vi "外设配置对话框.vi"() -> ()   [LabVIEW 2016, in "斯坦道氟化物.lvlib"]
uses:
  <vilib>/Utility/miscctls.llb/LVPointTypeDef.ctl
panel:
  out "选项卡控件":enum32{"V3 A版", "V3 B版"}(tab)
  in  "A版外设配置":T1 {"阀方向" items=["顺时针", "逆时针", "就近"]; "总氮x公式0" items=["0", "1"]; "光谱仪类型" items=["1型", "2型", "3型", "2型氙灯联控"]; "泵阀量" items=["9通"=9, "10通"=10, "12通"=12]; "泵类型" items=["1型", "2型", "sy04型+旋转阀"]}
  in  "B版外设配置":T2 {"阀型号" items=["垦拓10通阀"]; "总氮x公式0" items=["0", "1"]; "光谱仪类型" items=["1型", "2型", "3型", "2型氙灯联控"]; "泵阀量" items=["9通"=9, "10通"=10, "12通"=12]; "泵类型" items=["润泽注射泵", "垦拓注射泵"]}
  in  "关闭":bool
  in  "保存":bool
  in  "读取":bool
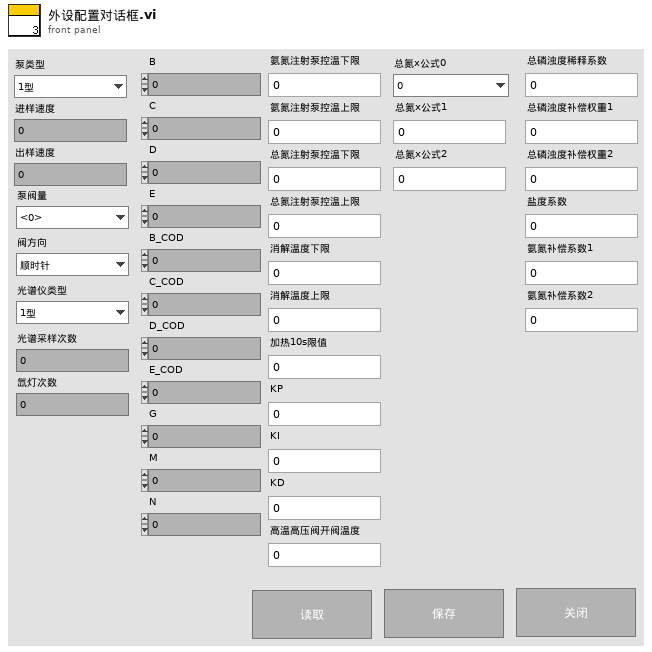
[diagram p1: front panel]
types:
  T1 = typedef "斯坦道氟化物.lvlib/V3 A版外设参数.ctl" = cluster{"泵类型":u8, "进样速度":u32, "出样速度":u32, "泵阀量":u8, "阀方向":u8, "光谱仪类型":u8, "光谱采样次数":u8, "氙灯次数":u8, "B":u16, "C":u16, "D":u16, "E":u16, "B_COD":u16, "C_COD":u16, "D_COD":u16, "E_COD":u16, "G":u16, "M":u16, "N":u16, "氨氮注射泵控温下限":sgl, "氨氮注射泵控温上限":sgl, "总氮注射泵控温下限":sgl, "总氮注射泵控温上限":sgl, "消解温度下限":sgl, "消解温度上限":sgl, "加热10s限值":sgl, "KP":sgl, "KI":sgl, "KD":sgl, "高温高压阀开阀温度":sgl, "总氮x公式0":u8, "总氮x公式1":sgl, "总氮x公式2":sgl, "总磷浊度稀释系数":sgl, "总磷浊度补偿权重1":sgl, "总磷浊度补偿权重2":sgl, "盐度系数":sgl, "氨氮补偿系数1":sgl, "氨氮补偿系数2":sgl}
  T2 = typedef "斯坦道氟化物.lvlib/V3 B版外设参数.ctl" = cluster{"泵类型":u8, "注射泵正常速度":u32, "注射泵慢速":u32, "泵阀量":u8, "阀型号":u8, "光谱仪类型":u8, "光谱采样次数":u8, "氙灯次数":u8, "B":u16, "C":u16, "D":u16, "E":u16, "B_COD":u16, "C_COD":u16, "D_COD":u16, "E_COD":u16, "G":u16, "M":u16, "N":u16, "氨氮注射泵控温下限":sgl, "氨氮注射泵控温上限":sgl, "总氮注射泵控温下限":sgl, "总氮注射泵控温上限":sgl, "消解温度下限":sgl, "消解温度上限":sgl, "加热10s限值":sgl, "KP":sgl, "KI":sgl, "KD":sgl, "高温高压阀开阀温度":sgl, "总氮x公式0":u8, "总氮x公式1":sgl, "总氮x公式2":sgl, "总磷浊度稀释系数":sgl, "总磷浊度补偿权重1":sgl, "总磷浊度补偿权重2":sgl, "盐度系数":sgl, "氨氮补偿系数1":sgl, "氨氮补偿系数2":sgl}
  T3 = typedef "LVPointTypeDef.ctl" = cluster{"Horizontal":i16, "Vertical":i16}
  T4 = typedef "调试控件V3.xctl/仪器类型.ctl" = enum16{"A版", "B版"}
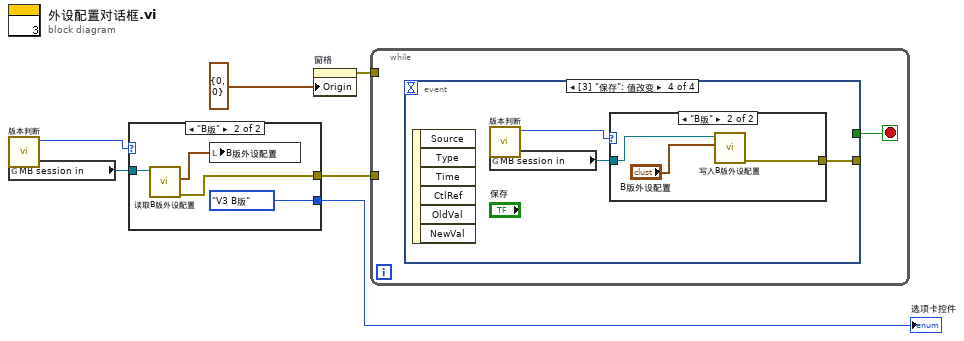
[diagram p0: block diagram]
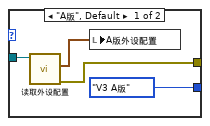
[diagram p2: hidden frame]
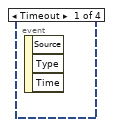
[diagram p3: hidden frame]
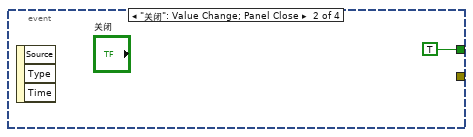
[diagram p4: hidden frame]
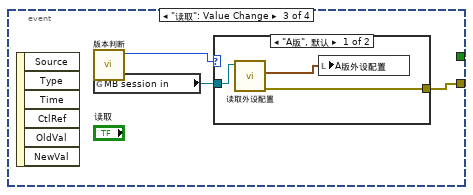
[diagram p5: hidden frame]
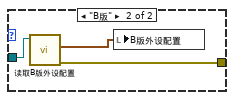
[diagram p6: hidden frame]
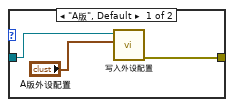
[diagram p7: hidden frame]
diagram:
  n1 = call "版本判断.vi"() -> ("仪器类型"=w3:T4)  [unwired: 11 in]
  n2 = global read "VAR总磷总氮全局变量.vi" "MB session in"() -> (w2:refnum<class "MB_Master.lvclass">)
  n3 = case shown="\"B版\"" w3 {
    tunnel: [w10 w13] -> w6
    tunnel: w2 -> [w8 w14]
    tunnel: [enum32{"V3 A版", "V3 B版"}."V3 A版" ("选项卡控件") enum32{"V3 A版", "V3 B版"}."V3 B版" ("选项卡控件")] -> w1
    frame "A版", Default {
      n4 = call "读取外设配置.vi"("MB session in"=w8) -> ("error out"=w10:errorcluster, "外设配置"=w9:T1)  [unwired: 8 in, 1 out]
      n5 = local write "A版外设配置"(w9) -> ()
    }
    frame "B版" {
      n6 = call "读取B版外设配置.vi"("MB session in"=w14) -> ("error out"=w13:errorcluster, "外设配置"=w12:T2)  [unwired: 8 in, 1 out]
      n7 = local write "B版外设配置"(w12) -> ()
    }
  }
  "选项卡控件" <- w1
  n8 = property on="窗格" class="Pane"("Origin"=T3 {"Horizontal"=0, "Vertical"=0} ("原点")) -> (error out=w4:errorcluster)  [unwired: 2 in, 1 out]
  n9 = while {
    tunnel: w6 -> [_]
    tunnel: w4 -> [_]
    stop <- w15 stop-if-true
    n10 = event shown="[3] \"保存\": 值改变" {
      selector: _ -> [_ _ _ _]
      dyn-events: _ -> [_ _ _ _]
      timeout: _ -> [_ _ _ _]
      tunnel: [_ TRUE _ _] -> w15
      tunnel: [_ _ w19 w28] -> _
      event Timeout {
        n11 = event-data() -> ()  [unwired: 1 in, 3 out]
      }
      event "关闭": Value Change; Panel Close {
        n12 = event-data() -> ()  [unwired: 1 in, 3 out]
      }
      event "读取": Value Change {
        n13 = event-data() -> ()  [unwired: 1 in, 6 out]
        n14 = call "版本判断.vi"() -> ("仪器类型"=w18:T4)  [unwired: 11 in]
        n15 = global read "VAR总磷总氮全局变量.vi" "MB session in"() -> (w17:refnum<class "MB_Master.lvclass">)
        n16 = case shown="\"A版\", 默认" w18 {
          tunnel: [w22 w24] -> w19
          tunnel: w17 -> [w20 w25]
          frame "A版", Default {
            n17 = call "读取外设配置.vi"("MB session in"=w20) -> ("error out"=w22:errorcluster, "外设配置"=w21:T1)  [unwired: 8 in, 1 out]
            n18 = local write "A版外设配置"(w21) -> ()
          }
          frame "B版" {
            n19 = call "读取B版外设配置.vi"("MB session in"=w25) -> ("error out"=w24:errorcluster, "外设配置"=w23:T2)  [unwired: 8 in, 1 out]
            n20 = local write "B版外设配置"(w23) -> ()
          }
        }
      }
      event "保存": Value Change {
        n21 = event-data() -> ()  [unwired: 1 in, 6 out]
        n22 = call "版本判断.vi"() -> ("仪器类型"=w26:T4)  [unwired: 11 in]
        n23 = global read "VAR总磷总氮全局变量.vi" "MB session in"() -> (w27:refnum<class "MB_Master.lvclass">)
        n24 = case shown="\"B版\"" w26 {
          tunnel: [w31 w32] -> w28
          tunnel: w27 -> [w30 w33]
          frame "A版", Default {
            n25 = call "写入外设配置.vi"("外设配置"="A版外设配置", "MB session in"=w30) -> ("error out"=w31:errorcluster)  [unwired: 8 in, 1 out]
          }
          frame "B版" {
            n26 = call "写入B版外设配置.vi"("外设配置"="B版外设配置", "MB session in"=w33) -> ("error out"=w32:errorcluster)  [unwired: 8 in, 1 out]
          }
        }
      }
    }
  }
